vi "Is Cluster.vi"(11 "Value":variant) -> (3 "Checkbox":bool)   [LabVIEW 2019]
uses:
  <vilib>/Utility/Data Type/NI_Data Type.lvlib
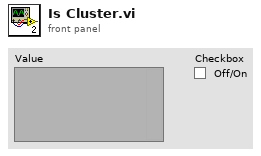
[diagram p1: front panel]
types:
  T1 = typedef "NI_Data Type.lvlib/Data Type.ctl" = enum8{"Invalid Type", "Void", "I8", "I16", "I32", "I64", "U8", "U16", "U32", "U64", "Single Float", "Double Float", "Extended Float", "Single Complex", "Double Complex", "Extended Complex", "Enum U8", "Enum U16", "Enum U32", "Enum U64", "Single Float With Unit", "Double Float With Unit", "Extended Float With Unit", "Single Complex with Unit", "Double Complex with Unit", "Extended Complex with Unit", "Boolean", "String", "Path", "Picture", "Tag", "Array", "Cluster", "Variant", "LV Variant", "Waveform", "Timestamp", "Digital Waveform", "Digital Data", "ExpressData", "Refnum", "External Data", "VI", "Poly VI", "LabVIEW Class Instance", "Fixed Point", "Set Collection", "Map Collection"}
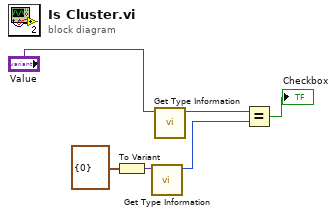
[diagram p0: block diagram]
diagram:
  n1 = To Variant(anything=cluster{i32} {0}) -> (Variant=w2:variant)
  n2 = call <vilib>:"Get Type Information.vi"("variant"=w2) -> ("type"=w4:T1)  [unwired: 6 in, 4 out]
  n3 = call <vilib>:"Get Type Information.vi"("variant"="Value") -> ("type"=w3:T1)  [unwired: 6 in, 4 out]
  n4 = Equal?(x=w3, y=w4) -> (x = y?=→"Checkbox":bool)
